vi "Configure Trigger.vi"   [LabVIEW 2015, in "Agilent 2000 3000 X-Series.lvlib"]
doc: "Configures trigger settings."
uses:
  <instrlib>/Agilent 2000 3000 X-Series/Agilent 2000 3000 X-Series.lvlib
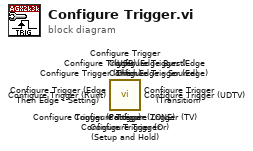
[diagram p0: block diagram]
diagram:
  n1 = call <instrlib>:"Configure Trigger (ZONE).vi"() -> ()  [unwired: 10 in, 2 out]
  n2 = call <instrlib>:"Configure Trigger (Edge Then Edge - Source).vi"() -> ()  [unwired: 10 in, 2 out]
  n3 = call <instrlib>:"Configure Trigger (Edge Then Edge - Setting).vi"() -> ()  [unwired: 10 in, 2 out]
  n4 = call <instrlib>:"Configure Trigger (UDTV).vi"() -> ()  [unwired: 10 in, 2 out]
  n5 = call <instrlib>:"Configure Trigger (Or).vi"() -> ()  [unwired: 10 in, 2 out]
  n6 = call <instrlib>:"Configure Trigger (Glitch).vi"() -> ()  [unwired: 10 in, 2 out]
  n7 = call <instrlib>:"Configure Trigger (USB).vi"() -> ()  [unwired: 10 in, 2 out]
  n8 = call <instrlib>:"Configure Trigger (TV).vi"() -> ()  [unwired: 10 in, 2 out]
  n9 = call <instrlib>:"Configure Trigger (Transition).vi"() -> ()  [unwired: 10 in, 2 out]
  n10 = call <instrlib>:"Configure Trigger (Setup and Hold).vi"() -> ()  [unwired: 10 in, 2 out]
  n11 = call <instrlib>:"Configure Trigger (Runt).vi"() -> ()  [unwired: 10 in, 2 out]
  n12 = call <instrlib>:"Configure Trigger (Pattern).vi"() -> ()  [unwired: 10 in, 2 out]
  n13 = call <instrlib>:"Configure Trigger (Edge).vi"() -> ()  [unwired: 10 in, 2 out]
  n14 = call <instrlib>:"Configure Trigger (Edge Burst).vi"() -> ()  [unwired: 10 in, 2 out]
